vi "Coerce image size.vi"(11 "Camera Parameters (important) in":T1={"Exposure Time (sec)"=0.0, "EM CCD Gain"=230, "Readout Settings"={"Acquisition Mode"=enum."Frame Transfer Run till Abort", "Pixel Rate"=enum."EM CCD 30 Mhz 16 bits", "High Capacity?"=FALSE, "V Shift Speed (us/row)"=enum."0.6 (not reccommended)", "V Shift Amplitude"=enum."normal", "Preamp Gain"=enum."2", "Trigger Mode"=0, "Baseline offset"=0, "Baseline clamp"=FALSE}, "Image Size"={"H Bin"=1, "V Bin"=1, "Left"=1, "Top"=1, "Right"=512, "Bottom"=512}} {"Readout Settings"."Baseline offset" min=-1000 max=1000 step=100; "Readout Settings"."Trigger Mode" items=["Internal", "External"]; "EM CCD Gain" scale=1.0..300.0; "Exposure Time (sec)" scale=0.001..10.0 scale format="%#_1g"}) -> (3 "Camera Parameters (important) out":T1={"Exposure Time (sec)"=0.0, "EM CCD Gain"=230, "Readout Settings"={"Acquisition Mode"=enum."(do not use)", "Pixel Rate"=enum."EM CCD 30 Mhz 16 bits", "High Capacity?"=FALSE, "V Shift Speed (us/row)"=enum."4.33", "V Shift Amplitude"=enum."normal", "Preamp Gain"=enum."2", "Trigger Mode"=0, "Baseline offset"=0, "Baseline clamp"=FALSE}, "Image Size"={"H Bin"=1, "V Bin"=1, "Left"=1, "Top"=1, "Right"=512, "Bottom"=512}} {"Readout Settings"."Baseline offset" min=-1000 max=1000 step=100; "Readout Settings"."Trigger Mode" items=["Internal", "External"]; "EM CCD Gain" scale=1.0..300.0; "Exposure Time (sec)" scale=0.001..10.0 scale format="%#_1g"})   [LabVIEW 2016]
uses:
  ixon ultra 897/HAL camera parameters important.ctt
  ixon ultra 897/ixon readout settings.ctl
  ixon ultra 897/andor acquisition mode.ctl
  ixon ultra 897/camera defaults globals.vi
panel:
  # "Camera: Andor iXon Ultra"
  # "Camera: Andor iXon Ultra"
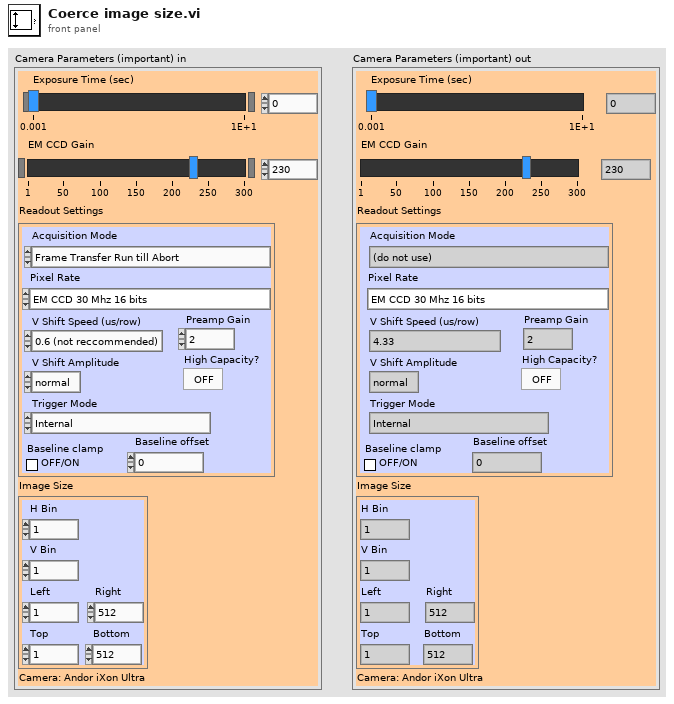
[diagram p1: front panel]
types:
  T1 = typedef "HAL camera parameters important.ctt" = cluster{"Exposure Time (sec)":sgl, "EM CCD Gain":u16, "Readout Settings":T2, "Image Size":cluster{"H Bin":i32, "V Bin":i32, "Left":i32, "Top":i32, "Right":i32, "Bottom":i32}}
  T2 = typedef "ixon readout settings.ctl" = cluster{"Acquisition Mode":T3, "Pixel Rate":enum16{"EM CCD 30 Mhz 16 bits", "EM CCD 20 Mhz 16 bits", "EM CCD 10 Mhz 16 bits", "EM CCD 1 Mhz 16 bits", "Standard CCD 1 Mhz 16 bits", "Standard CCD 0.1 Mhz 16 bits"}, "High Capacity?":bool, "V Shift Speed (us/row)":enum16{"0.6 (not reccommended)", "1.13  (not reccommended)", "2.2  (not reccommended)", "4.33"}, "V Shift Amplitude":enum16{"normal", "+1", "+2", "+3", "+4"}, "Preamp Gain":enum16{"1", "2", "3"}, "Trigger Mode":u32, "Baseline offset":i16, "Baseline clamp":bool}
  T3 = typedef "andor acquisition mode.ctl" = enum16{"(do not use)", "Single Scan", "Accumulate", "Kinetics", "Fast Kinetics", "Kinetics Run till Abort", "Frame Transfer", "Frame Transfer Run till Abort", "(do not use) ", "Time Delayed Integration"}
  T4 = typedef "image size.ctl" = cluster{"H Bin":i32, "V Bin":i32, "Left":i32, "Top":i32, "Right":i32, "Bottom":i32}
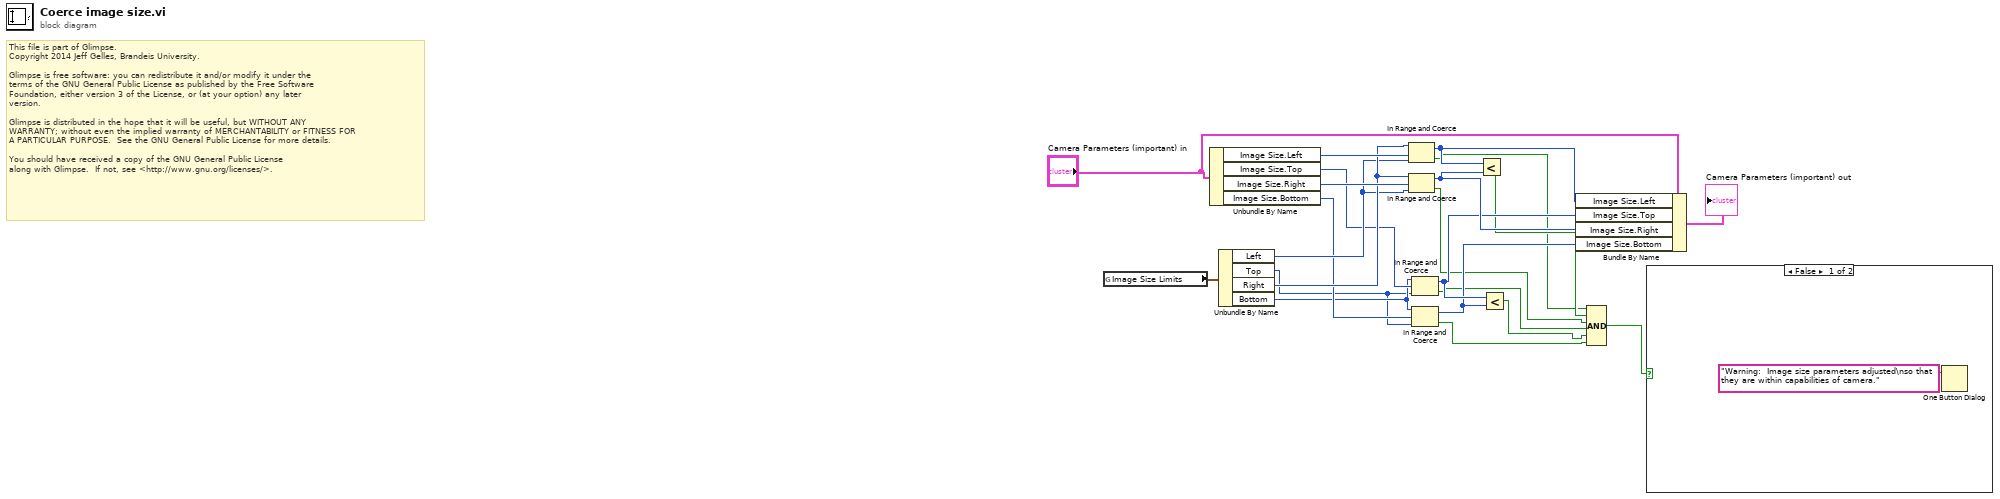
[diagram p0: block diagram]
diagram:
  # "This file is part of Glimpse. \nCopyright 2014 Jeff Gelles, Brandeis University.    \n\nGlimpse is free software: you can redistribute it and/or modify it under the \nterms of the GNU General Public License as published by the Free Software \nFoundation, either version 3 of the License, or (at your option) any later \nversion.\n\nGlimpse is distributed in the hope that it will be useful, but WITHOUT ANY \nWARRANTY; without even the implied warranty of MERCHANTABILITY or FITNESS FOR \nA PARTICULAR PURPOSE.  See the GNU General Public License for more details.\n\nYou should have received a copy of the GNU General Public License\nalong with Glimpse.  If not, see <http://www.gnu.org/licenses/>."
  n1 = global read "camera defaults globals.vi" "Image Size Limits"() -> (w22:T4)
  n2 = Unbundle By Name("Camera Parameters (important) in") -> ("Image Size.Left"=w21:i32, "Image Size.Top"=w13:i32, "Image Size.Right"=w20:i32, "Image Size.Bottom"=w12:i32)
  n3 = Unbundle By Name(w22) -> ("Left"=w18:i32, "Top"=w10:i32, "Right"=w19:i32, "Bottom"=w11:i32)
  n4 = In Range and Coerce(upper limit=w19, x=w21, lower limit=w18) -> (coerced(x)=w15:i32, In Range?=w2:bool)
  n5 = In Range and Coerce(upper limit=w19, x=w20, lower limit=w18) -> (coerced(x)=w14:i32, In Range?=w4:bool)
  n6 = In Range and Coerce(upper limit=w11, x=w13, lower limit=w10) -> (coerced(x)=w9:i32, In Range?=w5:bool)
  n7 = In Range and Coerce(upper limit=w11, x=w12, lower limit=w10) -> (coerced(x)=w8:i32, In Range?=w7:bool)
  n8 = Less?(x=w15, y=w14) -> (x < y?=w3:bool)
  n9 = Less?(x=w9, y=w8) -> (x < y?=w6:bool)
  n10 = Bundle By Name(cluster="Camera Parameters (important) in", "Image Size.Left"=w15, "Image Size.Top"=w9, "Image Size.Right"=w14, "Image Size.Bottom"=w8) -> (→"Camera Parameters (important) out":T1)
  n11 = Compound Arithmetic op=AND(w2, w3, w4, w5, w6, w7) -> (w1:bool)
  n12 = case shown="False" w1 {
    frame False {
      n13 = One Button Dialog(message="Warning:  Image size parameters adjusted\nso that they are within capabilities of camera.") -> ()  [unwired: 1 in, 1 out]
    }
    frame True {
    }
  }
